vi "HeadPos(SubVI).vi"(8 "error in (no error)":errorcluster, 10 "VISA resource name":refnum<visa-resource-name>="GPIB0::11::INSTR", 11 "Checkbox":bool) -> (0 "error out":errorcluster, 2 "VISA resource name 2":refnum<visa-resource-name>)   [LabVIEW 2020]
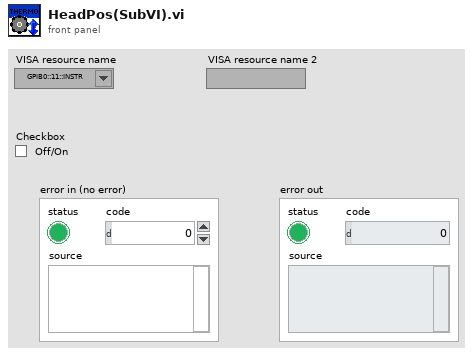
[diagram p1: front panel]
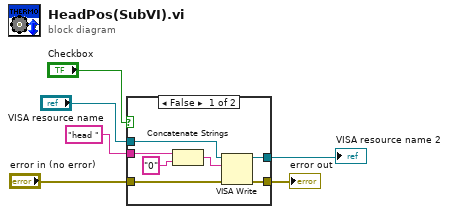
[diagram p0: block diagram]
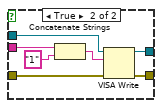
[diagram p2: hidden frame]
diagram:
  n1 = case shown="False" "Checkbox" {
    tunnel: [w8 w20] -> w1
    tunnel: [w7 w19] -> w6
    tunnel: "VISA resource name" -> [w11 w18]
    tunnel: "error in (no error)" -> [w10 w17]
    tunnel: "head " ("write buffer") -> [w9 w16]
    frame False {
      n2 = Concatenate Strings(w9, "0" ("string")) -> (w13:string)
      n3 = VISA Write(VISA resource name=w11, write buffer=w13, error in (no error)=w10) -> (VISA resource name out=w8:refnum<visa-resource-name>, error out=w7:errorcluster)  [unwired: 1 out]
    }
    frame True {
      n4 = Concatenate Strings(w16, "1" ("string")) -> (w15:string)
      n5 = VISA Write(VISA resource name=w18, write buffer=w15, error in (no error)=w17) -> (VISA resource name out=w20:refnum<visa-resource-name>, error out=w19:errorcluster)  [unwired: 1 out]
    }
  }
  "error out" <- w6
  "VISA resource name 2" <- w1
